vi "QTrkFreeAllTrackers.vi"   [LabVIEW 2011]
uses:
  QTrkDLL.vi
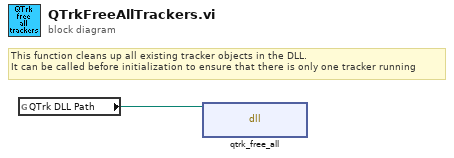
[diagram p0: block diagram]
diagram:
  # "This function cleans up all existing tracker objects in the DLL.\nIt can be called before initialization to ensure that there is only one tracker running"
  n1 = global read "QTrkDLL.vi" "QTrk DLL Path"() -> (w1:path)
  n2 = dll-call lib="D:/jcnossen1/cudaqi-tracker/bin/jtrk-labview.dll" fn="qtrk_free_all"(path in=w1) -> ()  [unwired: 3 in, 2 out]
